vi "find_peak_frequency (SubVI).vi"(1 "Signal":dbl[](array[numeric])) -> (0 "Frequency":dbl)   [LabVIEW 2012]
uses:
  <vilib>/Analysis/NI_AALPro.lvlib
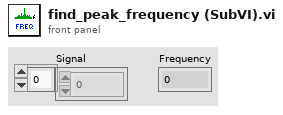
[diagram p1: front panel]
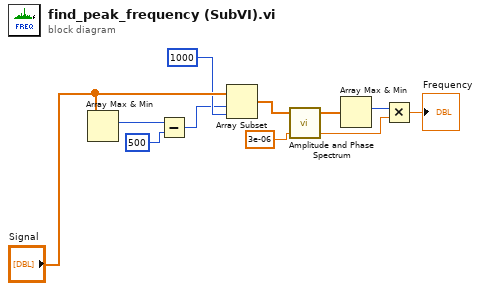
[diagram p0: block diagram]
diagram:
  n1 = Array Max & Min(array="Signal") -> (max index (indices)=w1:i32)  [unwired: 3 out]
  n2 = Subtract(x=w1, y=500) -> (x-y=w3:i32)
  n3 = Array Subset(array="Signal", index=w3, length=1000) -> (w5:dbl[])
  n4 = call <vilib>:"Amplitude and Phase Spectrum.vi"("dt"=3e-06, "Signal (V)"=w5) -> ("df"=w9:dbl, "Amp Spectrum Mag (Vrms)"=w6:dbl[])  [unwired: 1 in, 1 out]
  n5 = Array Max & Min(array=w6) -> (max index (indices)=w7:i32)  [unwired: 3 out]
  n6 = Multiply(x=w7, y=w9) -> (x*y=→"Frequency":dbl)
